vi "update listbox with streams.vi"(7 "MulticolumnListbox in":refnum<vi>, 8 "error in (no error)":errorcluster, 11 "Item Ref in":T1 format="%.0x") -> (0 "error out":errorcluster)   [LabVIEW 2026, in "Nominal Core Streaming System Explorer.lvlib"]
uses:
  Nominal Core Streaming System Explorer.lvlib
  <vilib>/NI VeriStand/Custom Device API/Custom Device API.lvlib
  Shared/Nominal Core Streaming Shared.lvlib
  <vilib>/NI VeriStand/Custom Device API/Custom Device Item Ref.ctl
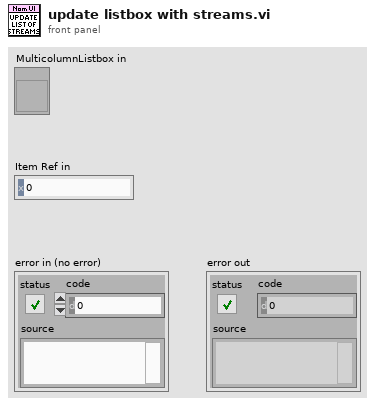
[diagram p1: front panel]
types:
  T1 = typedef "Custom Device API.lvlib/Custom Device Item Ref.ctl" = u64
  T2 = typedef "Custom Device API.lvlib/Custom Device Item Info.ctl" = cluster{"Name":string, "Is Channel":bool, "GUID":string, "Is Waveform":bool}
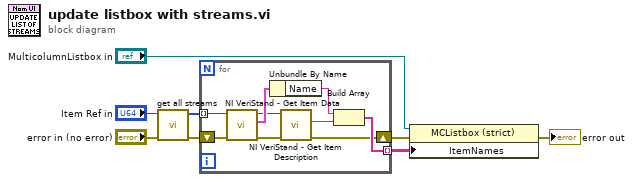
[diagram p0: block diagram]
diagram:
  n1 = call "get all streams.vi"("error in (no error)"="error in (no error)", "CD in"="Item Ref in") -> ("error out"=w2:errorcluster, "streams"=w1:T1[])  [unwired: 8 in]
  n2 = for {
    tunnel: w1 -> [w16] mode=indexing
    tunnel: [w12] -> w3 mode=indexing
    shift-right: [w11] -> w4
    shift-left: w2 -> [w17]
    n3 = call <vilib>:"NI VeriStand - Get Item Data.vi"("error in (no error)"=w17, "Item Ref in"=w16) -> ("error out"=w9:errorcluster, "Item Info"=w15:T2, "Item Ref out"=w10:T1)  [unwired: 6 in, 1 out]
    n4 = Unbundle By Name(w15) -> ("Name"=w14:string)
    n5 = call <vilib>:"NI VeriStand - Get Item Description.vi"("error in (no error)"=w9, "Item Ref in"=w10) -> ("error out"=w11:errorcluster, "Description"=w13:string)  [unwired: 6 in, 2 out]
    n6 = Build Array(w14, w13) -> (w12:string[])
  }
  n7 = property on="Property Node" class="MCListbox (strict)"(reference="MulticolumnListbox in", error in=w4, "ItemNames"=w3) -> (error out=→"error out":errorcluster)  [unwired: 1 out]
